vi "global.vi"() -> ()   [LabVIEW 2023]
panel:
  out "stop":bool
  out "tablica bitów":bool[](array[boolean])
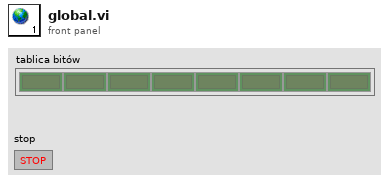
[diagram p1: front panel]
diagram:
